vi "Do.vi"(8 "error in (no error)":errorcluster, 10 "Actor in":refnum<class "Actor.lvclass">, 11 "TCP Command Received Msg":refnum<class "TCP Command Received Msg.lvclass">) -> (0 "error out":errorcluster, 2 "Actor out":refnum<class "Actor.lvclass">)   [LabVIEW 2013, in "tWorkerController.lvlib" / "TCP Command Received Msg.lvclass"]
doc: "(<B>Filename</B>: Actor Framework.lvlib:Message.lvclass:Do.vi)\n\nDefines what a message does when it is received by an actor. Generally, a message instructs an actor to invoke one of its methods.\n\nBy default, this method does nothing. A child class must override it to define behavior. Create a child class by using the Actor Framework Message Maker dialog box."
uses:
  TCP Command Received Msg.lvclass
  <vilib>/ActorFramework/Actor/Actor.lvclass
  tWorkerController/tWorkerController.lvclass
  TCP Command Received Msg.lvclass/TCP Command Received Msg.ctl
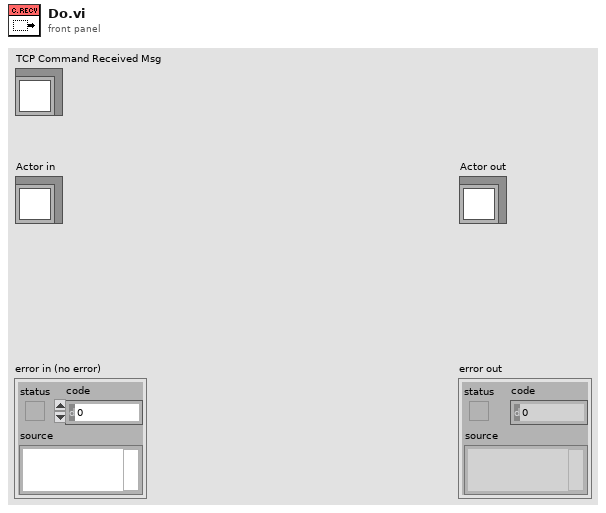
[diagram p1: front panel]
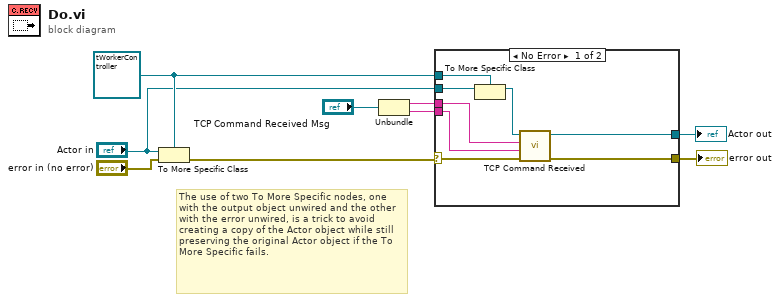
[diagram p0: block diagram]
diagram:
  w8 = refnum<class "tWorkerController.lvclass"> refnum ("Actor in")
  # "The use of two To More Specific nodes, one with the output object unwired and the other with the error unwired, is a trick to avoid creating a copy of the Actor object while still preserving the original Actor object if the To More Specific fails."
  n1 = To More Specific Class(target class=w8, reference="Actor in", error in="error in (no error)") -> (error out=w9:errorcluster)  [unwired: 1 out]
  n2 = Unbundle("TCP Command Received Msg") -> (w7:string, w6:string)
  n3 = case shown="No Error" w9 {
    selector: w9 -> [w12 w19]
    tunnel: [w13 w19] -> w1
    tunnel: [w14 w18] -> w2
    tunnel: "Actor in" -> [w17 w18]
    tunnel: w8 -> [w16 _]
    tunnel: w7 -> [w11 _]
    tunnel: w6 -> [w10 _]
    frame No Error {
      n4 = To More Specific Class(target class=w16, reference=w17) -> (specific class reference=w15:refnum<class "tWorkerController.lvclass">)  [unwired: 1 in, 1 out]
      n5 = call "TCP Command Received.vi"("error in (no error)"=w12, "Message"=w10, "GUID"=w11, "tWorkerController in"=w15) -> ("error out"=w13:errorcluster, "tWorkerController out"=w14:refnum<class "tWorkerController.lvclass">)  [unwired: 6 in]
    }
    frame Error {
      # "If type check fails, pass the original object out again."
    }
  }
  "error out" <- w1
  "Actor out" <- w2
